vi "Report Generator.vi"(8 "error in (no error)":errorcluster, 11 "Report Generator In":refnum<class "Report Generator.lvclass">) -> (0 "error out":errorcluster)   [LabVIEW 2020, in "Reports.lvlib" / "Report Generator.lvclass"]
uses:
  Report Generator.lvclass
  C:/git/astemes-lunit/source/User Interface/Process/Process.lvclass
  User Interface/Process/Process.lvclass/Process.ctl
  Report Generator.lvclass/Report Generator.ctl
  <vilib>/Platform/browser.llb/Open URL in Default Browser (path).vi
  Framework/Report Interface/Report Interface.lvclass
  User Interface/Process/Process.lvclass
  User Interface/Support/Paths.lvlib
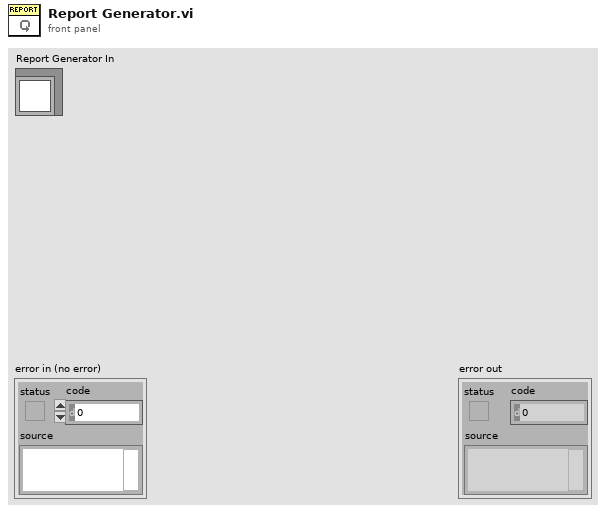
[diagram p1: front panel]
types:
  T1 = typedef "Result.lvlib/Result.ctl" = cluster{"Name":string, "Description":string, "Status":T2, "Result Type":T3, "Execution Time":dbl, "Data":cluster{"Expected":variant, "Actual":variant, "Delta":variant}}
  T2 = typedef "Result.lvlib/Status.ctl" = enum16{"", "Passed", "Failed", "Error", "Skipped", "Setup Error", "Broken", "Teardown Error"}
  T3 = typedef "Result.lvlib/Type.ctl" = enum16{"Test Case", "Test Suite", "Test Run", "Pass", "Fail", "Skip", "Pass if", "Fail if", "Pass if Error", "Fail if Error", "Pass if Equal", "Fail if Equal"}
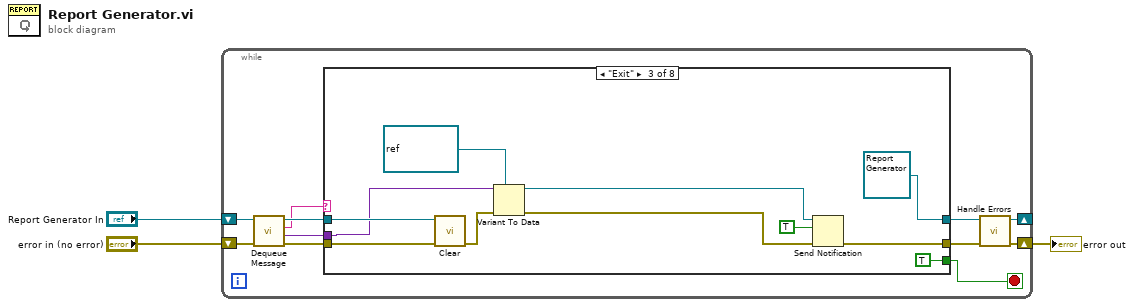
[diagram p0: block diagram]
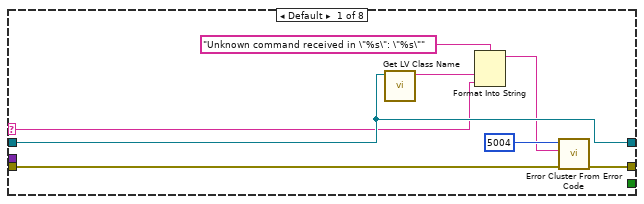
[diagram p2: hidden frame]
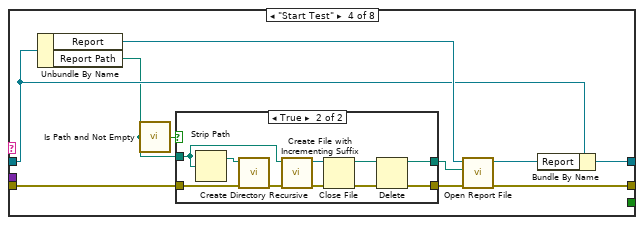
[diagram p4: hidden frame]
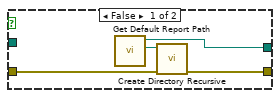
[diagram p5: hidden frame]
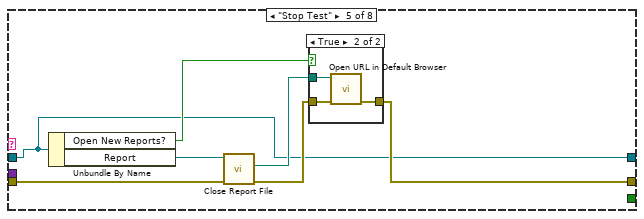
[diagram p6: hidden frame]
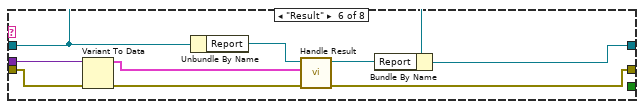
[diagram p8: hidden frame]
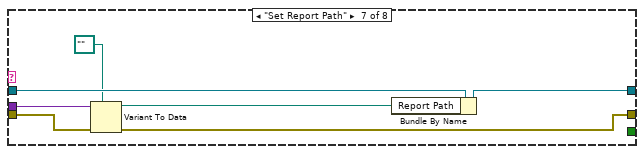
[diagram p9: hidden frame]
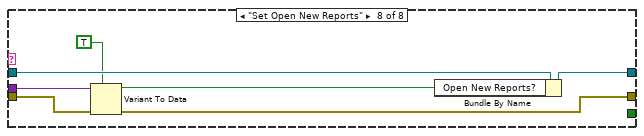
[diagram p10: hidden frame]
diagram:
  n1 = while {
    shift-right: [w6] -> w1
    shift-left: "error in (no error)" -> [w13]
    shift-right: [w8] -> _
    shift-left: "Report Generator In" -> [w11]
    stop <- w7 stop-if-true
    n2 = call "Dequeue Message.vi"("error in (no error)"=w13, "Process In"=w11) -> ("error out"=w12:errorcluster, "Message Data"=w10:variant, "Message"=w5:string, "Process Out"=w9:refnum<class "Report Generator.lvclass">)  [unwired: 6 in]
    n3 = case shown="\"Exit\"" w5 {
      selector: w5 -> [w18 _ _ _ _ _ _ _]
      tunnel: w12 -> [w21 w22 w32 w36 w65 w78 w85 w92]
      tunnel: [w20 w22 w30 w44 w63 w77 w80 w89] -> w4
      tunnel: w10 -> [_ _ w29 _ _ w75 w82 w88]
      tunnel: w9 -> [w19 w23 w33 w40 w59 w71 w84 w91]
      tunnel: [w19 w23 refnum<class "Report Generator.lvclass"> refnum ("Process Out") w42 w59 w72 w83 w90] -> w8
      tunnel: [_ _ TRUE _ _ _ _ _] -> w7
      frame Default {
        n4 = call <vilib>:"Get LV Class Name.vi"("object"=w19) -> ("class name"=w17:string)  [unwired: 9 in, 1 out]
        n5 = Format Into String(format string="Unknown command received in \"%s\": \"%s\"", w17, w18) -> (resulting string=w14:string)  [unwired: 2 in, 1 out]
        n6 = call <vilib>:"Error Cluster From Error Code.vi"("error in (no error)"=w21, "error message (\"\")"=w14, "error code (0)"=5004) -> ("error out"=w20:errorcluster)  [unwired: 6 in]
      }
      frame "Init" {
      }
      frame "Exit" {
        n7 = call-dynamic "Clear.vi"("error in (no error)"=w32, "Process In"=w33) -> ("error out"=w27:errorcluster)  [unwired: 9 in]
        n8 = Variant To Data(error in=w27, type=refnum<notifier> refnum ("notifier out"), Variant=w29) -> (data=w25:refnum<notifier>, error out=w26:errorcluster)
        n9 = Send Notification(notification=TRUE, notifier=w25, error in (no error)=w26) -> (error out=w30:errorcluster)  [unwired: 1 out]
      }
      frame "Start Test" {
        n10 = Unbundle By Name(w40) -> ("Report"=w43:refnum<class "Report Interface.lvclass">, "Report Path"=w39:path)
        n11 = call <vilib>:"Is Path and Not Empty.vi"("path"=w39) -> ("Is Path and Not Empty?"=w35:bool)  [unwired: 4 in]
        n12 = case shown="True" w35 {
          tunnel: w39 -> [_ w55]
          tunnel: [w48 w51] -> w37
          tunnel: w36 -> [w47 w52]
          tunnel: [w46 w49] -> w38
          frame False {
            n13 = call "Get Default Report Path.vi"() -> ("Default Report Directory"=w45:path, "Default Report Path"=w46:path)  [unwired: 10 in]
            n14 = call <vilib>:"Create Directory Recursive.vi"("error in (no error)"=w47, "directory"=w45) -> ("error out"=w48:errorcluster)  [unwired: 3 in, 2 out]
          }
          frame True {
            n15 = Strip Path(path=w55) -> (stripped path=w54:path)  [unwired: 1 out]
            n16 = call <vilib>:"Create Directory Recursive.vi"("error in (no error)"=w52, "directory"=w54) -> ("error out"=w53:errorcluster)  [unwired: 3 in, 2 out]
            n17 = call <vilib>:"Create File with Incrementing Suffix.vi"("error in (no error)"=w53, "file path"=w55) -> ("error out"=w56:errorcluster, "refnum out"=w57:refnum<file>)  [unwired: 7 in, 1 out]
            n18 = Close File(refnum=w57, error in=w56) -> (path=w50:path, error out=w58:errorcluster)
            n19 = Delete(path (use dialog)=w50, error in=w58) -> (deleted path=w49:path, error out=w51:errorcluster)  [unwired: 3 in, 1 out]
          }
        }
        n20 = call-dynamic "Open Report File.vi"("error in (no error)"=w37, "Path"=w38, "Report Interface In"=w43) -> ("error out"=w44:errorcluster, "Report Interface Out"=w41:refnum<class "Report Interface.lvclass">)  [unwired: 7 in]
        n21 = Bundle By Name(cluster=w40, "Report"=w41) -> (w42:refnum<class "Report Generator.lvclass">)
      }
      frame "Stop Test" {
        n22 = Unbundle By Name(w59) -> ("Open New Reports?"=w62:bool, "Report"=w60:refnum<class "Report Interface.lvclass">)
        n23 = call-dynamic "Close Report File.vi"("error in (no error)"=w65, "Report Interface In"=w60) -> ("error out"=w64:errorcluster, "Report Path"=w61:path)  [unwired: 8 in]
        n24 = case shown="True" w62 {
          tunnel: w61 -> [_ w67]
          tunnel: w64 -> [w66 w69]
          tunnel: [w66 w68] -> w63
          frame False {
          }
          frame True {
            n25 = call-poly <vilib>:"Open URL in Default Browser.vi"("error in (no error)"=w69, "path"=w67) -> ("error out"=w68:errorcluster)  [unwired: 4 in, 1 out]
          }
        }
      }
      frame "Result" {
        n26 = Variant To Data(error in=w78, Variant=w75) -> (data=w74:T1, error out=w76:errorcluster)  [unwired: 1 in]
        n27 = Unbundle By Name(w71) -> ("Report"=w73:refnum<class "Report Interface.lvclass">)
        n28 = call-dynamic "Handle Result.vi"("error in (no error)"=w76, "Result"=w74, "Report in"=w73) -> ("error out"=w77:errorcluster, "Report out"=w70:refnum<class "Report Interface.lvclass">)  [unwired: 7 in]
        n29 = Bundle By Name(cluster=w71, "Report"=w70) -> (w72:refnum<class "Report Generator.lvclass">)
      }
      frame "Set Report Path" {
        n30 = Variant To Data(error in=w85, type=path "", Variant=w82) -> (data=w79:path, error out=w80:errorcluster)
        n31 = Bundle By Name(cluster=w84, "Report Path"=w79) -> (w83:refnum<class "Report Generator.lvclass">)
      }
      frame "Set Open New Reports" {
        n32 = Variant To Data(error in=w92, type=TRUE, Variant=w88) -> (data=w87:bool, error out=w89:errorcluster)
        n33 = Bundle By Name(cluster=w91, "Open New Reports?"=w87) -> (w90:refnum<class "Report Generator.lvclass">)
      }
    }
    n34 = call "Handle Errors.vi"("error in (no error)"=w4) -> ("error out"=w6:errorcluster)  [unwired: 10 in]
  }
  "error out" <- w1
